vi "GetHierarchyItemByChildPath.vi"(8 "error in (no error)":errorcluster, 9 "Child ILabVIEWItem":refnum<class "ILabVIEWItem.lvclass">, 11 "CDependencyList in":refnum<class "CDependencyList.lvclass">) -> (0 "error out":errorcluster, 1 "Hierarchy items":refnum<class "ILabVIEWItem.lvclass">[](array[class]), 3 "CDependencyList out":refnum<class "CDependencyList.lvclass">)   [LabVIEW 2020, in "DependencyInspection.lvlib" / "CDependencyList.lvclass"]
uses:
  CDependencyList.lvclass
  obj/Addons/LabVIEWObjectInterfaces.lvlibp/LabVIEWObjectInterfaces/ILabVIEWItem/ILabVIEWItem.lvclass
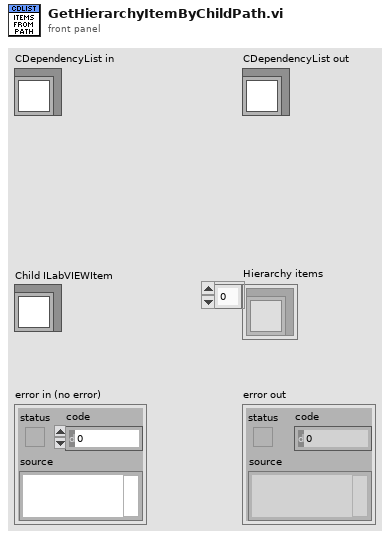
[diagram p1: front panel]
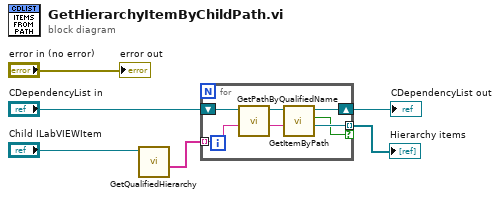
[diagram p0: block diagram]
diagram:
  n1 = call-dynamic "GetQualifiedHierarchy.vi"("ILabVIEWItem in"="Child ILabVIEWItem") -> ("Qualified hierarchy"=w5:string[])  [unwired: 8 in, 2 out]
  n2 = for {
    shift-right: [w13] -> w4
    shift-left: "CDependencyList in" -> [w11]
    tunnel: w5 -> [w9] mode=indexing
    tunnel: [w12] -> w3 mode=indexing if=w7
    n3 = call-dynamic "GetPathByQualifiedName.vi"("Qualified name"=w9, "CDependencyList in"=w11) -> ("Path"=w8:string, "CDependencyList out"=w10:refnum<class "CDependencyList.lvclass">)  [unwired: 6 in, 2 out]
    n4 = call-dynamic "GetItemByPath.vi"("Path"=w8, "CDependencyList in"=w10) -> ("ILabVIEWItem"=w12:refnum<class "ILabVIEWItem.lvclass">, "key found?"=w7:bool, "CDependencyList out"=w13:refnum<class "CDependencyList.lvclass">)  [unwired: 6 in, 1 out]
  }
  "CDependencyList out" <- w4
  "Hierarchy items" <- w3
  "error out" <- "error in (no error)"
